vi "Change Icon Text to Project Name.vi"(8 "error in":errorcluster, 10 "Overlay Icon":refnum<class "Icon.lvclass">, 11 "Lvclass Ref in":refnum<vi>) -> (0 "error out":errorcluster, 2 "Layer.lvclass out":refnum<class "Layer.lvclass">, 3 "Lvclass Ref out":refnum<vi>, 5 "Body Text.Line 1 text":string)   [LabVIEW 2023, in "Plugin Generator.lvlib"]
uses:
  Plugin Generator.lvlib
  <vilib>/LabVIEW Icon API/lv_icon/Classes/Layer/Layer.lvclass
  <vilib>/LabVIEW Icon API/lv_icon/Classes/Icon/Icon.lvclass
  <vilib>/LabVIEW Icon API/lv_icon/Controls/Layer.ctl
  <vilib>/LabVIEW Icon API/LabVIEW Icon API.lvlib
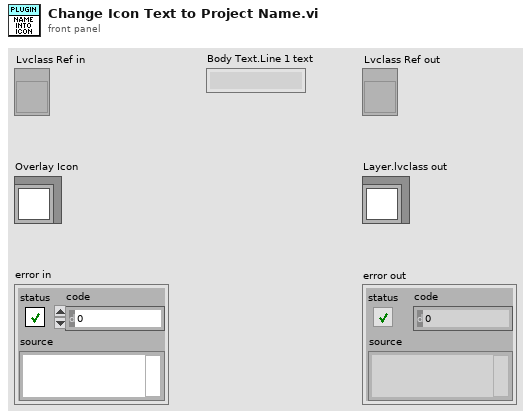
[diagram p1: front panel]
types:
  T1 = typedef "Layer.ctl" = cluster{"LayerIcon":picture, "LayerName":string, "Opacity":u8, "Visibility?":bool}
  T2 = typedef "imagedata.ctl" = cluster{"image type":i32, "image depth":i32, "image":u8[], "mask":u8[], "colors":u32[], "Rectangle":cluster{"left":i16, "top":i16, "right":i16, "bottom":i16}}
  T3 = typedef "LabVIEW Icon Stored Information.ctl" = cluster{"Text Visible?":bool, "Text Opacity":u8, "Templ Visible?":bool, "Templ Opacity":u8, "Relative Path from 1 to 2":path, "Image":picture, "All User Layers":refnum<class "Layer.lvclass">[], "Body Text":T4}
  T4 = typedef "BodyText.ctl" = cluster{"Line 1 text":string, "Line 2 text":string, "Line 3 text":string, "Line 4 text":string, "Line 1 color":u32, "Line 2 color":u32, "Line 3 color":u32, "Line 4 color":u32, "Body Text Spec":cluster{"Font":T5, "Alignment":T6, "Size":u8}, "Center text vertically":bool, "Capitalize Text":bool}
  T5 = typedef "Font.ctl" = string
  T6 = typedef "Alignment.ctl" = u16
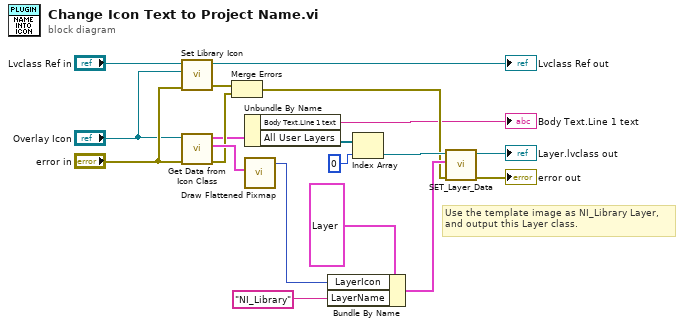
[diagram p0: block diagram]
diagram:
  # "Use the template image as NI_Library Layer,\nand output this Layer class."
  n1 = call <vilib>:"Set Library Icon.vi"("error in (no error)"="error in", "Icon"="Overlay Icon", "Library Refnum in"="Lvclass Ref in") -> ("error out"=w14:errorcluster, "Library Refnum out"=→"Lvclass Ref out":refnum<vi>)  [unwired: 7 in]
  n2 = call <vilib>:"Get Data from Icon Class.vi"("error in (no error)"="error in", "Icon in"="Overlay Icon") -> ("error out"=w15:errorcluster, "Color Image Data"=w19:T2, "Icon data"=w7:T3)  [unwired: 6 in, 1 out]
  n3 = Merge Errors(w14, w15) -> (w5:errorcluster)
  n4 = Unbundle By Name(w7) -> ("Body Text.Line 1 text"=→"Body Text.Line 1 text":string, "All User Layers"=w13:refnum<class "Layer.lvclass">[])
  n5 = call <vilib>:"Draw Flattened Pixmap.vi"("image data"=w19) -> ("new picture"=w8:picture)  [unwired: 8 in]
  n6 = Bundle By Name(cluster=T1 {"LayerIcon"=bytes[3102], "LayerName"="", "Opacity"=100, "Visibility?"=TRUE} ("Data"), "LayerIcon"=w8, "LayerName"="NI_Library") -> (w11:T1)
  n7 = Index Array(array=w13, index=0) -> (element=w6:refnum<class "Layer.lvclass">)
  n8 = call-dynamic "SET_Layer_Data.vi"("error in (no error)"=w5, "Data"=w11, "Layer.lvclass in"=w6) -> ("error out"=→"error out":errorcluster, "Layer.lvclass out"=→"Layer.lvclass out":refnum<class "Layer.lvclass">)  [unwired: 7 in]
